vi "cálculo npr y dr.vi"(4 "Numeric Control":i32, 6 ">>d>>":dbl[](array[numeric]), 7 "Numeric Control 2":i32, 9 ">>n[]>>":csg[](array[numeric]), 10 ">>lambda>>":dbl, 11 ">>nsr>>":cdb[](array[numeric])) -> (2 ">>dr>>":cdb[](array[numeric]), 3 ">>nPr>>":csg[](array[numeric]))   [LabVIEW 2025]
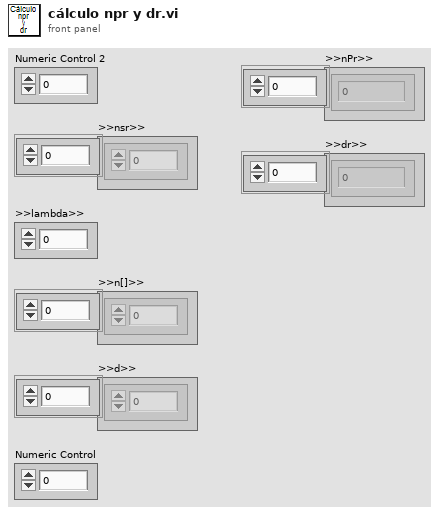
[diagram p1: front panel]
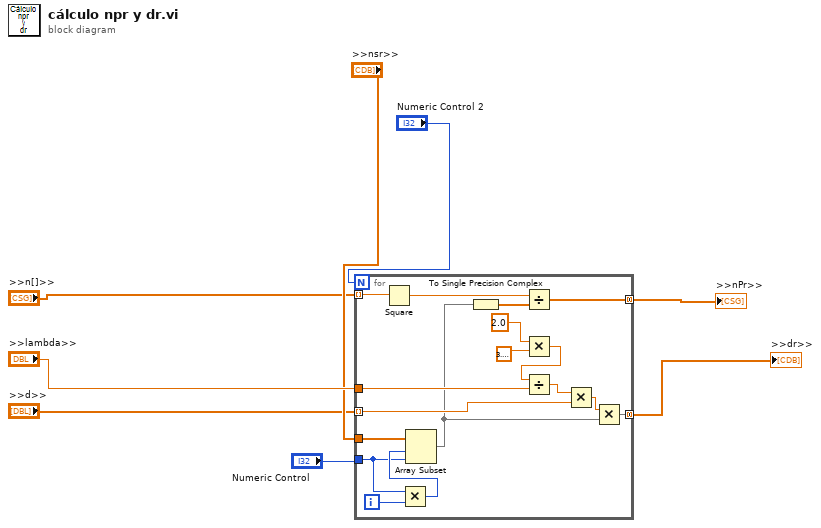
[diagram p0: block diagram]
diagram:
  n1 = for {
    N: "Numeric Control 2" -> [_]
    tunnel: ">>d>>" -> [w12] mode=indexing
    tunnel: ">>n[]>>" -> [w25] mode=indexing
    tunnel: ">>nsr>>" -> [w24]
    tunnel: [w20] -> w8 mode=concatenating
    tunnel: "Numeric Control" -> [w18]
    tunnel: ">>lambda>>" -> [w14]
    tunnel: [w9] -> w7 mode=concatenating
    i -> [w23]
    n2 = Square(x=w25) -> (x^2=w21:csg)
    n3 = Multiply(x=w18, y=w23) -> (x*y=w22:i32)
    n4 = Array Subset(array=w24, index=w22, length=w18) -> (w10:cdb[])
    n5 = To Single Precision Complex(1:w10) -> (0:w19:csg[])
    n6 = Divide(x=w21, y=w19) -> (x/y=w20:csg[])
    n7 = Multiply(x=2.0, y=3.141592653589793) -> (x*y=w15:dbl)
    n8 = Divide(x=w15, y=w14) -> (x/y=w13:dbl)
    n9 = Multiply(x=w13, y=w12) -> (x*y=w11:dbl)
    n10 = Multiply(x=w11, y=w10) -> (x*y=w9:cdb[])
  }
  ">>nPr>>" <- w8
  ">>dr>>" <- w7
